vi "Etape2.vi"() -> ()   [LabVIEW 2020]
uses:
  <instrlib>/Agilent 34401/Public/Data/Read (Single Point).vi
  <instrlib>/Agilent E363X Series/Agilent E363X Series.lvlib
  <instrlib>/Agilent 34401/Agilent 34401.lvlib
panel:
  out "XY Graph":cluster{"Y":dbl[], "Y":dbl[]}[](graph) caption="Graphe XY"
  in  "Plage tension":dbl(slide) scale=0.0..6.0
  out "Courant":dbl
  in  "Incrément tension":dbl
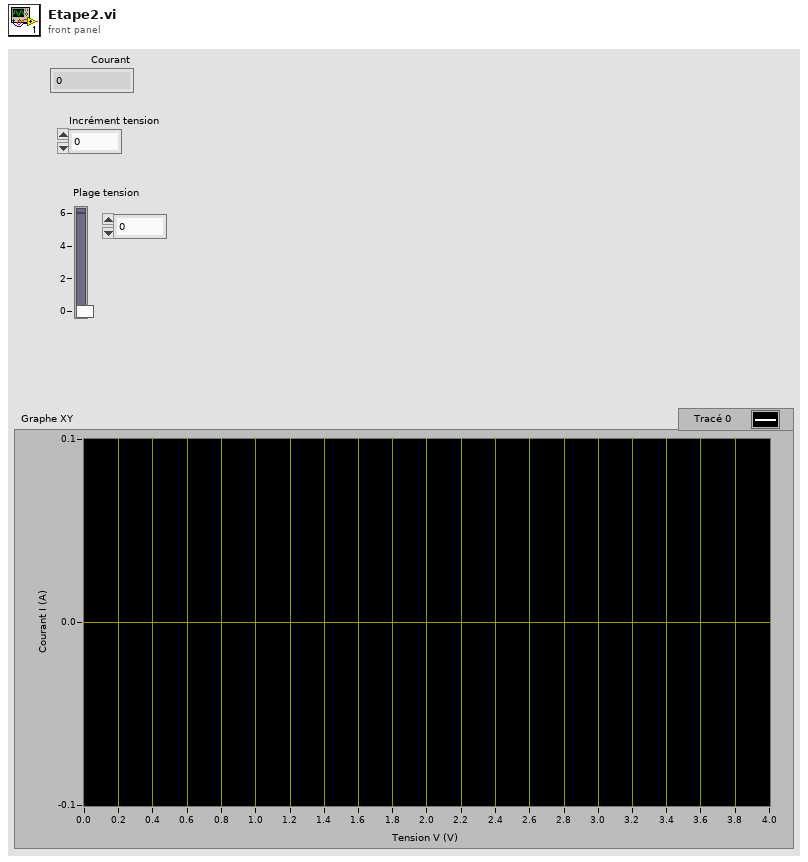
[diagram p1: front panel]
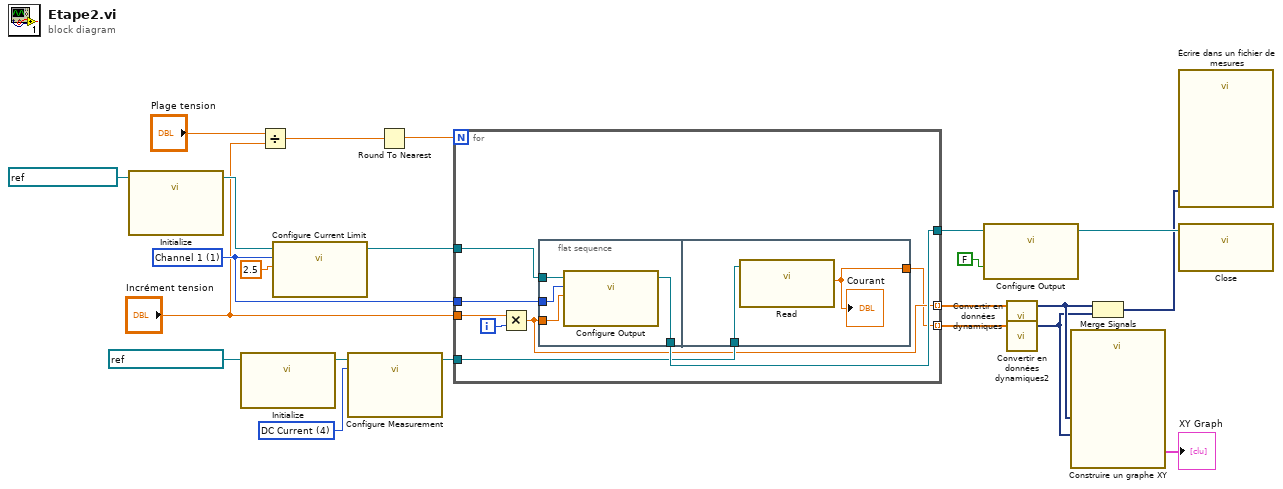
[diagram p0: block diagram]
diagram:
  w17 = u16 4 items=["DC Voltage", "AC Voltage", "2 - Wire Resistance", "4 - Wire Resistance", "DC Current", "AC Current", "Frequency", "Period", "Continuity", "Diode Checking", "VDC:VDC Ratio", "Temperature", "Capacitance"] ("Function (0: DC Voltage)")
  w13 = 1 items=["Channel 1"=1, "Channel 2"=2, "Channel 3"=3] ("Channel (1: Channel 1)")
  n1 = call <instrlib>:"Initialize.vi"("VISA resource name"=refnum<visa-resource-name> "GPIB0::5::INSTR" ("VISA resource name out")) -> ("VISA resource name out"=w22:refnum<visa-resource-name>)  [unwired: 9 in, 1 out]
  n2 = call <instrlib>:"Initialize.vi"("VISA resource name"=refnum<visa-resource-name> "GPIB0::22::INSTR") -> ("VISA resource name out"=w18:refnum<visa-resource-name>)  [unwired: 9 in, 1 out]
  n3 = Divide(x="Plage tension", y="Incrément tension") -> (x/y=w9:dbl)
  n4 = call <instrlib>:"Configure Current Limit.vi"("Current Limit (0.0 A)"=2.5, "Channel (1: Channel 1)"=w13, "VISA resource name"=w22) -> ("VISA resource name out"=w12:refnum<visa-resource-name>)  [unwired: 7 in, 1 out]
  n5 = call <instrlib>:"Configure Measurement.vi"("Function (0: DC Voltage)"=w17, "VISA resource name"=w18) -> ("VISA resource name out"=w14:refnum<visa-resource-name>)  [unwired: 8 in, 1 out]
  n6 = Round To Nearest(number=w9) -> (nearest integer value=w7:dbl)
  n7 = for {
    N: w7 -> [_]
    tunnel: w14 -> [w27]
    tunnel: w13 -> [w30]
    tunnel: w12 -> [w29]
    tunnel: [w28] -> w11
    tunnel: "Incrément tension" -> [w26]
    tunnel: [w24] -> w5 mode=indexing
    tunnel: [w23] -> w4 mode=indexing
    i -> [w25]
    n8 = Multiply(x=w26, y=w25) -> (x*y=w24:dbl)
    n9 = flat-sequence {
      tunnel: w30 -> [w34]
      tunnel: w29 -> [w33]
      tunnel: [w32] -> w28
      tunnel: w24 -> [w31]
      tunnel: w27 -> [w36]
      tunnel: [w35] -> w23
      frame #0 {
        n10 = call <instrlib>:"Configure Output.vi"("Voltage Level (0.0 V)"=w31, "Channel (1: Channel 1)"=w34, "VISA resource name"=w33) -> ("VISA resource name out"=w32:refnum<visa-resource-name>)  [unwired: 7 in, 1 out]
      }
      frame #1 {
        n11 = call-poly <instrlib>:"Read.vi"("VISA resource name"=w36) -> ("Measurement"=w35:dbl)  [unwired: 8 in, 2 out]
        "Courant" <- w35
      }
    }
  }
  n12 = call <instrlib>:"Configure Output.vi"("Enable Output (T: Enable)"=FALSE, "VISA resource name"=w11) -> ("VISA resource name out"=w15:refnum<visa-resource-name>)  [unwired: 8 in, 1 out]
  n13 = call "Convertir en données dynamiques"("Array"=w5) -> ("Dynamic Data Type"=w3:dynamicdata)  [unwired: 3 in]
  n14 = call "Convertir en données dynamiques2"("Array"=w4) -> ("Dynamic Data Type"=w2:dynamicdata)  [unwired: 3 in]
  n15 = call "Construire un graphe XY"("Y Input"=w2, "X Input"=w3) -> ("XY Graph"=→"XY Graph":cluster{"X":dbl[], "Y":dbl[]}[])  [unwired: 8 in, 1 out]
  n16 = Merge Signals(w3, w2) -> (w1:dynamicdata)
  n17 = call "Écrire dans un fichier de mesures"("Signals"=w1) -> ()  [unwired: 16 in, 3 out]
  n18 = call <instrlib>:"Close.vi"("VISA resource name"=w15) -> ()  [unwired: 10 in, 1 out]
